vi "Recieve Acknowledge Initialized.vi"(8 "error in (no error)":errorcluster, 9 "Requestor":string, 10 "Requestee":string, 11 "Compound Measurement in":refnum<class "Compound Measurement.lvclass">) -> (0 "error out":errorcluster, 3 "Compound Measurement out":refnum<class "Compound Measurement.lvclass">)   [LabVIEW 2015, in "Compound Measurement.lvclass"]
uses:
  Compound Measurement.lvclass
  Mag Lab Root/Mag Lab Root.lvclass/Mag Lab Root.ctl
  Compound Measurement.lvclass/Compound Measurement.ctl
  <vilib>/ActorFramework/Actor/Actor.lvclass/Actor.ctl
  <vilib>/ActorFramework/Message Enqueuer/Message Enqueuer.lvclass/Message Enqueuer.ctl
  Mag Lab Root Messages/Recieve Acknowledge Initialized Msg/Recieve Acknowledge Initialized Msg.lvclass/Recieve Acknowledge Initialized Msg.ctl
  Mag Lab Root/Read Original requestor.vi
  <vilib>/ActorFramework/Message Enqueuer/Init from Existing Queue.vi
  <vilib>/ActorFramework/Message Enqueuer/Enqueue.vi
  <vilib>/ActorFramework/Message Priority Queue/Priority Enqueue.vi
  <vilib>/ActorFramework/Message Enqueuer/Message Enqueuer.lvclass
  Mag Lab Root Messages/Recieve Acknowledge Initialized Msg/Recieve Acknowledge Initialized Msg.lvclass
  Mag Lab Root/Mag Lab Root.lvclass
  <vilib>/ActorFramework/Actor/Actor.lvclass
  Mag Lab Error Handler/Mag Lab Error Handler.lvclass
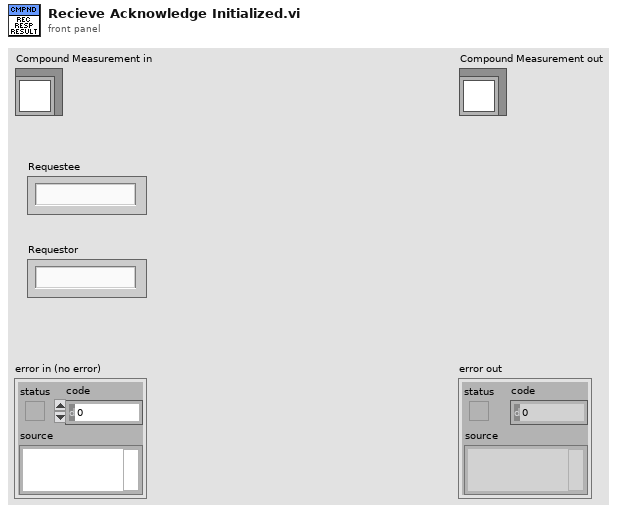
[diagram p1: front panel]
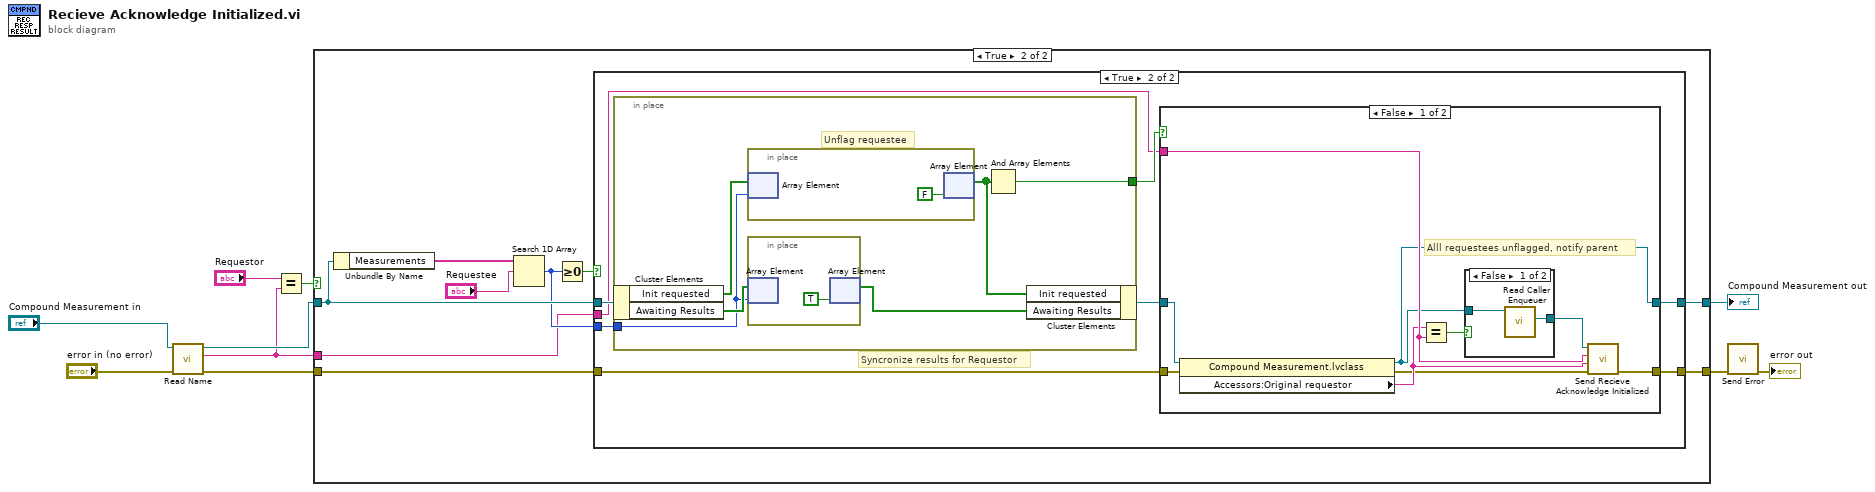
[diagram p0: block diagram]
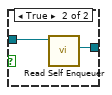
[diagram p4: hidden frame]
diagram:
  n1 = call "Read Name.vi"("error in (no error)"="error in (no error)", "Mag Lab Root in"="Compound Measurement in") -> ("error out"=w3:errorcluster, "Name"=w4:string, "Mag Lab Root out"=w8:refnum<class "Compound Measurement.lvclass">)  [unwired: 7 in]
  n2 = Equal?(x="Requestor", y=w4) -> (x = y?=w9:bool)
  n3 = case shown="True" w9 {
    tunnel: w8 -> [w12 w19]
    tunnel: [w12 w17] -> w7
    tunnel: w4 -> [_ w15]
    tunnel: [w11 w14] -> w2
    tunnel: w3 -> [w11 w13]
    frame False {
    }
    frame True {
      n4 = Unbundle By Name(w19) -> ("Measurements"=w21:string[])
      n5 = Search 1D Array(1D array=w21, element="Requestee") -> (index of element=w18:i32)  [unwired: 1 in]
      n6 = Greater Or Equal To 0?(x=w18) -> (x >= 0?=w16:bool)
      n7 = case shown="True" w16 {
        tunnel: w19 -> [w23 w31]
        tunnel: w18 -> [_ w30]
        tunnel: [w23 w26] -> w17
        tunnel: w15 -> [_ w27]
        tunnel: [w22 w25] -> w14
        tunnel: w13 -> [w22 w24]
        frame False {
        }
        frame True {
          # "Syncronize results for Requestor"
          n8 = in-place {
            in-place-border: w30 -> [w48]
            in-place-border: [w50] -> w29
            # "Unflag requestee"
            n9 = in-place-cluster #1(w31) -> ("Init requested"=w52:bool[], "Awaiting Results"=w49:bool[])
            n10 = in-place {
              n11 = in-place-array #2(w52, w48) -> ()  [unwired: 1 out]
              n12 = in-place-array #2(FALSE ("new element/subarray")) -> (w51:bool[])  [unwired: 1 out]
            }
            n13 = in-place {
              n14 = in-place-array #3(w49, w48) -> ()  [unwired: 1 out]
              n15 = in-place-array #3(TRUE ("new element/subarray")) -> (w47:bool[])  [unwired: 1 out]
            }
            n16 = And Array Elements(Boolean array=w51) -> (logical AND=w50:bool)
            n17 = in-place-cluster #1("Init requested"=w51, "Awaiting Results"=w47) -> (w28:refnum<class "Compound Measurement.lvclass">)
          }
          n18 = case shown="False" w29 {
            tunnel: w28 -> [w38 w46]
            tunnel: w27 -> [w37 _]
            tunnel: [w35 w46] -> w26
            tunnel: [w39 w45] -> w25
            tunnel: w24 -> [w33 w45]
            frame False {
              # "Alll requestees unflagged, notify parent"
              n19 = property class="Compound Measurement.lvclass"(reference=w38, error in=w33) -> (reference out=w35:refnum<class "Compound Measurement.lvclass">, error out=w32:errorcluster, "Accessors:Original requestor"=w34:string)
              n20 = Equal?(x=w34, y=w37) -> (x = y?=w36:bool)
              n21 = case shown="False" w36 {
                tunnel: [w42 w44] -> w40
                tunnel: w35 -> [w41 w43]
                frame False {
                  n22 = call <vilib>:"Read Caller Enqueuer.vi"("Actor"=w41) -> ("Caller Enqueuer"=w42:refnum<class "Message Enqueuer.lvclass">)  [unwired: 10 in]
                }
                frame True {
                  n23 = call <vilib>:"Read Self Enqueuer.vi"("Actor"=w43) -> ("Self Enqueuer"=w44:refnum<class "Message Enqueuer.lvclass">)  [unwired: 10 in]
                }
              }
              n24 = call "Send Recieve Acknowledge Initialized.vi"("error in (no error)"=w32, "Requestor"=w34, "Requestee"=w37, "Message Enqueuer"=w40) -> ("error out"=w39:errorcluster)  [unwired: 6 in, 1 out]
            }
            frame True {
            }
          }
        }
      }
    }
  }
  "Compound Measurement out" <- w7
  n25 = call "Send Error.vi"("error in (no error)"=w2) -> ("error out"=→"error out":errorcluster)  [unwired: 9 in, 1 out]
